vi "Example 1.vi"   [LabVIEW 2018]
uses:
  <vilib>/addons/VeriStand Custom Device Scripting APIs/FPGA Addon/Private/Import Bitfile Scalars (Instances)/Import Scalars - all.vi
  <vilib>/addons/VeriStand Custom Device Scripting APIs/FPGA Addon/Scripting API.lvlib
types:
  T1 = typedef "Custom Device API.lvlib/Custom Device Item Ref.ctl" = u64
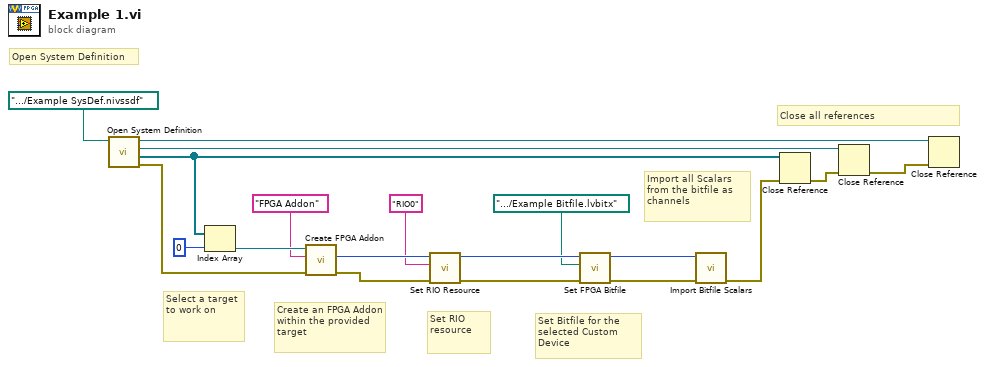
[diagram p0: block diagram]
diagram:
  # "Close all references"
  # "Import all Scalars from the bitfile as channels"
  # "Set Bitfile for the selected Custom Device"
  # "Set RIO resource"
  # "Create an FPGA Addon within the provided target"
  # "Select a target to work on"
  # "Open System Definition"
  n1 = call <vilib>:"Open System Definition.vi"("System Definition File"=path ".../Example SysDef.nivssdf" ("fpga bitfile path")) -> ("error out"=w16:errorcluster, "targets refnums"=w4:refnum<k24>[], "root refnum"=w5:refnum<k24>, "system definition refnum"=w6:refnum<k24>)  [unwired: 7 in]
  n2 = Index Array(array=w4, index=0) -> (element=w18:refnum<k24>)
  n3 = call <vilib>:"Create FPGA Addon.vi"("error in (no error)"=w16, "fpga addon name"="FPGA Addon", "target in"=w18) -> ("error out"=w14:errorcluster, "fpga addon refnum"=w15:T1)  [unwired: 6 in, 1 out]
  n4 = call <vilib>:"Set RIO Resource.vi"("error in (no error)"=w14, "rio resource in"="RIO0", "fpga addon refnum in"=w15) -> ("error out"=w12:errorcluster, "fpga addon refnum out"=w11:T1)  [unwired: 7 in]
  n5 = call <vilib>:"Set FPGA Bitfile.vi"("error in (no error)"=w12, "fpga bitfile path"=path ".../Example Bitfile.lvbitx", "fpga addon refnum in"=w11) -> ("error out"=w8:errorcluster, "fpga addon refnum out"=w7:T1)  [unwired: 7 in]
  n6 = call-poly <vilib>:"Import Bitfile Scalars.vi"("error in (no error)"=w8, "fpga addon refnum in"=w7) -> ("error out"=w3:errorcluster)  [unwired: 7 in, 2 out]
  n7 = Close Reference(reference=w4, error in (no error)=w3) -> (error out=w2:errorcluster)
  n8 = Close Reference(reference=w5, error in (no error)=w2) -> (error out=w1:errorcluster)
  n9 = Close Reference(reference=w6, error in (no error)=w1) -> ()  [unwired: 1 out]
